vi "PXIe-4139 Read Data Decision (RT).vi"(9 "Read Trigger Index":i32, 10 "Continuous Read? Index":i32, 11 "Array In":dbl[](array[numeric])) -> (3 "Read Data?":bool)   [LabVIEW 2023, in "PXIe-4139 Custom Device.lvlib"]
uses:
  PXIe-4139 Custom Device.lvlib
  <vilib>/ptbypt/NI_PtbyPt.lvlib
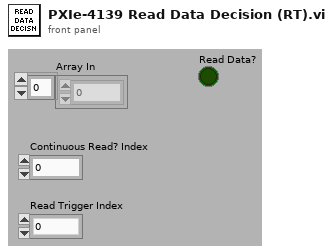
[diagram p1: front panel]
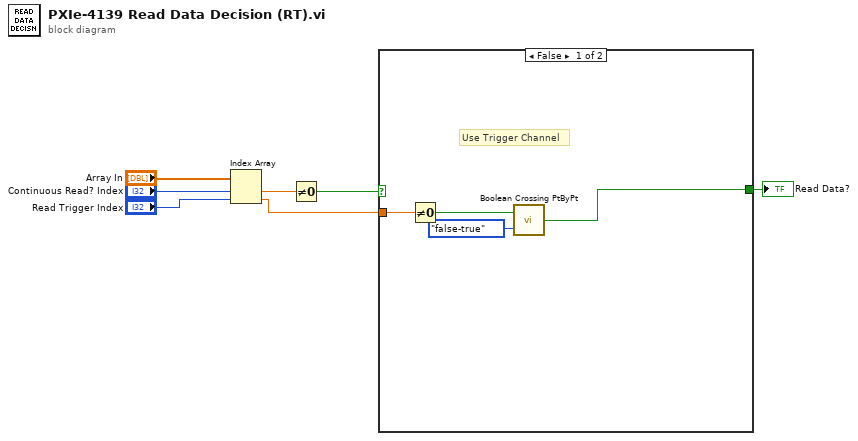
[diagram p0: block diagram]
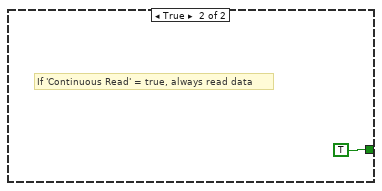
[diagram p2: hidden frame]
diagram:
  n1 = Index Array(array="Array In", index #1="Continuous Read? Index", index #2="Read Trigger Index") -> (element #1=w4:dbl, element #2=w1:dbl)
  n2 = Not Equal To 0?(x=w4) -> (x != 0?=w3:bool)
  n3 = case shown="False" w3 {
    tunnel: [w8 TRUE] -> w2
    tunnel: w1 -> [w9 _]
    frame False {
      # "Use Trigger Channel"
      n4 = Not Equal To 0?(x=w9) -> (x != 0?=w10:bool)
      n5 = call <vilib>:"Boolean Crossing PtByPt.vi"("direction"=enum16{"either", "false-true", "true-false"}."false-true", "input"=w10) -> ("crossing"=w8:bool)  [unwired: 1 in]
    }
    frame True {
      # "If 'Continuous Read' = true, always read data"
    }
  }
  "Read Data?" <- w2
